vi "SCM2 init.vi"(2 "Magnet ID":i32(ring) items=["None", "Cell 12", "Cell 15", "Cell 15insert", "Cell 4", "Cell 4-2", "Cell 4-3", "Cell 5", "Cell 6", "Cell 6-2", "Cell 6-3", "Cell 7", "Cell 8", "Cell 9", "Outsert", "SCM1", "SCM2"], 4 "Keithley GPIB Address":refnum<visa-resource-name>) -> (0 "Calibration":T1, 1 "Keithley GPIB output":refnum<visa-resource-name>)   [LabVIEW 2021]
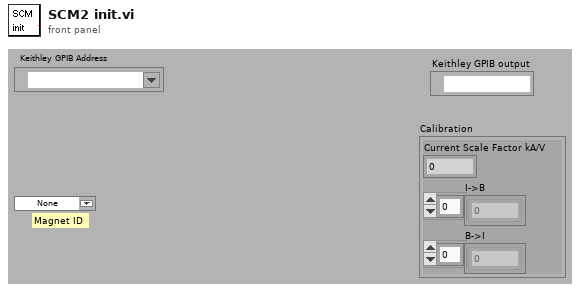
[diagram p1: front panel]
types:
  T1 = cluster{"Current Scale Factor kA/V":dbl, "I->B":dbl[], "B->I":dbl[]}
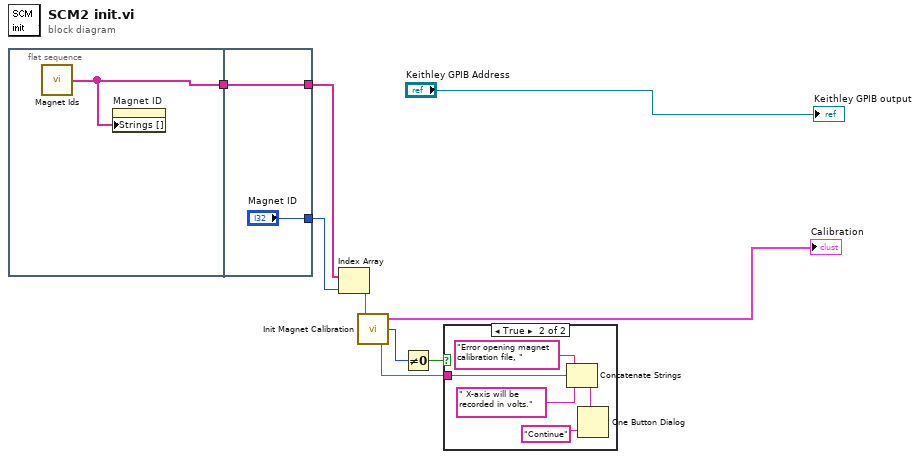
[diagram p0: block diagram]
diagram:
  n1 = flat-sequence {
    tunnel: [w10] -> w2
    tunnel: ["Magnet ID"] -> w3
    tunnel: [w11] -> w1
    tunnel: w2 -> [w11]
    frame #0 {
      n2 = call "Magnet Ids.vi"() -> ("Magnet IDs"=w10:string[])
      n3 = property on="Magnet ID" class="Ring (strict)"("Strings []"=w10) -> ()  [unwired: 2 in, 2 out]
    }
    frame #1 {
    }
  }
  n4 = Index Array(array=w1, index=w3) -> (element=w7:string)
  n5 = call "Init Magnet Calibration.vi"("Magnet Id"=w7) -> ("Calibration"=→"Calibration":T1, "Error Code"=w5:i32, "Error message"=w6:string)
  n6 = Not Equal To 0?(x=w5) -> (x != 0?=w4:bool)
  n7 = case shown="True" w4 {
    tunnel: w6 -> [_ w13]
    frame False {
    }
    frame True {
      n8 = Concatenate Strings("Error opening magnet calibration file, ", w13, " X-axis will be recorded in volts.") -> (w15:string)
      n9 = One Button Dialog(message=w15, button name ("OK")="Continue") -> ()  [unwired: 1 out]
    }
  }
  "Keithley GPIB output" <- "Keithley GPIB Address"
